vi "Create_Scan_comment_string.vi"(1 "Requested channels":i32[](array[numeric]), 2 "Scan comments":string[](array[string])) -> (0 "Comment string":string)   [LabVIEW 2010]
uses:
  ADAM_Global.vi
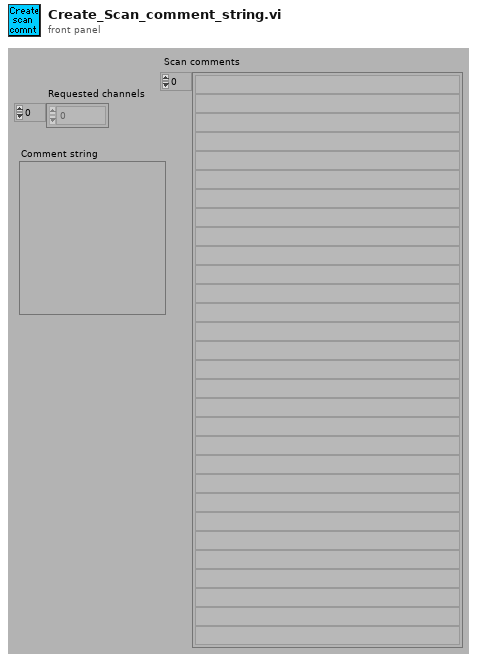
[diagram p1: front panel]
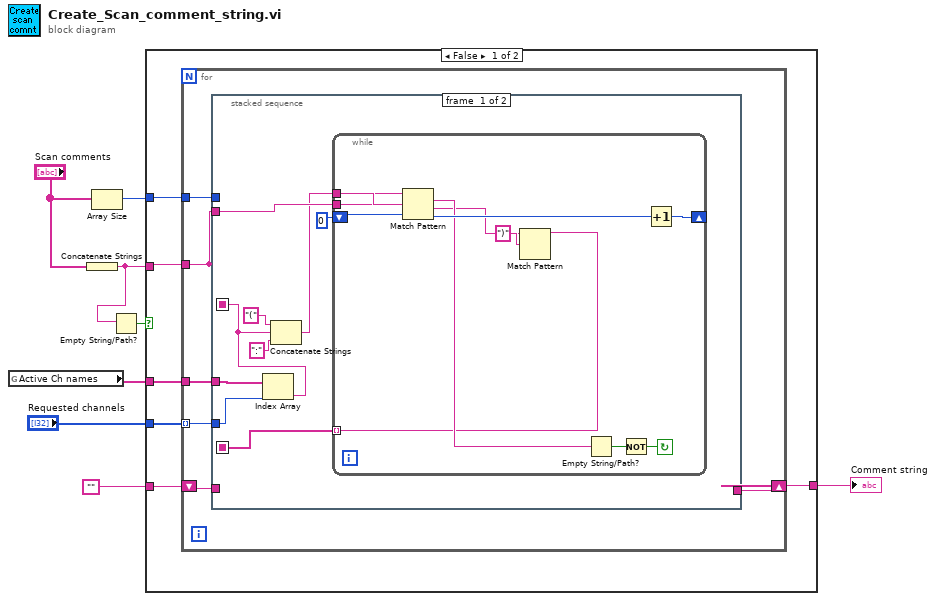
[diagram p0: block diagram]
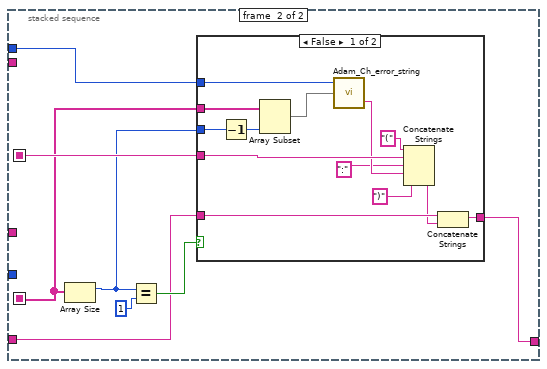
[diagram p2: hidden frame]
diagram:
  n1 = global read "ADAM_Global.vi" "Active Ch names"() -> (w7:string[])
  n2 = Concatenate Strings("Scan comments") -> (w4:string)
  n3 = Array Size(array="Scan comments") -> (size(s)=w1:i32)
  n4 = Empty String/Path?(string/path=w4) -> (empty?=w3:bool)
  n5 = case shown="False" w3 {
    tunnel: "Requested channels" -> [w14 _]
    tunnel: w7 -> [w13 _]
    tunnel: [w12 w63] -> w6
    tunnel: "" -> [w11 w63]
    tunnel: w4 -> [w10 _]
    tunnel: w1 -> [w9 _]
    frame False {
      n6 = for {
        tunnel: w14 -> [w20] mode=indexing
        tunnel: w13 -> [w19]
        tunnel: [w18] -> _ mode=indexing
        shift-right: [w16] -> w12
        shift-left: w11 -> [w17]
        tunnel: w10 -> [w18]
        tunnel: w9 -> [w15]
        n7 = stacked-sequence {
          seq-local: [w24 _] -> [_ w44]
          seq-local: [w22 _] -> [_ w42]
          tunnel: w20 -> [w21 _]
          tunnel: w19 -> [w29 _]
          tunnel: w18 -> [w28 _]
          tunnel: w17 -> [_ w46]
          tunnel: [_ w45] -> w16
          tunnel: w15 -> [_ w43]
          frame #0 {
            n8 = Index Array(array=w29, index=w21) -> (element=w24:string)
            n9 = Concatenate Strings("(", w24, ":") -> (w23:string)
            n10 = while {
              tunnel: [w30] -> w22 mode=indexing
              shift-left: 0 ("offset past match") -> [w34]
              shift-right: [w35] -> _
              tunnel: w28 -> [w39]
              tunnel: w23 -> [w40]
              stop <- w36 continue-if-true
              n11 = Match Pattern(string=w39, regular expression=w40, offset (0)=w34) -> (match substring=w32:string, after substring=w31:string, offset past match=w38:i32)  [unwired: 1 out]
              n12 = Match Pattern(string=w31, regular expression=")" ("String to match")) -> (before substring=w30:string)  [unwired: 4 out]
              n13 = Empty String/Path?(string/path=w32) -> (empty?=w37:bool)
              n14 = Not(x=w37) -> (.not. x?=w36:bool)
              n15 = Increment(x=w38) -> (x+1=w35:i32)
            }
          }
          frame #1 {
            n16 = Array Size(array=w42) -> (size(s)=w41:i32)
            n17 = Equal?(x=w41, y=1) -> (x = y?=w47:bool)
            n18 = case shown="False" w47 {
              tunnel: w44 -> [w60 _]
              tunnel: w46 -> [w59 w62]
              tunnel: [w57 w62] -> w45
              tunnel: w43 -> [w53 _]
              tunnel: w42 -> [w50 _]
              tunnel: w41 -> [w49 _]
              frame False {
                n19 = Decrement(x=w49) -> (x-1=w52:i32)
                n20 = Array Subset(array=w50, length=w52) -> (w51:string[])  [unwired: 1 in]
                n21 = call "Adam_Ch_error_string.vi"("String array"=w51, "Number of scans"=w53) -> ("Comment string"=w56:string)  [unwired: 2 out]
                n22 = Concatenate Strings("(", w60, ":", w56, ")") -> (w58:string)
                n23 = Concatenate Strings(w59, w58) -> (w57:string)
              }
              frame True {
              }
            }
          }
        }
      }
    }
    frame True {
    }
  }
  "Comment string" <- w6
